vi "Fibonacci - String.vi"(7 "Memo":string[](array[string]), 11 "n":u32) -> (3 "fib(n)":string)   [LabVIEW 2013, in "Problem 25.lvlib"]
uses:
  Problem 25.lvlib
  Problem 20/Problem 20.lvlib
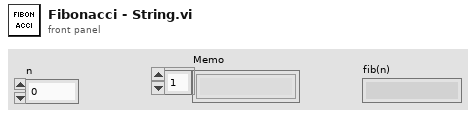
[diagram p1: front panel]
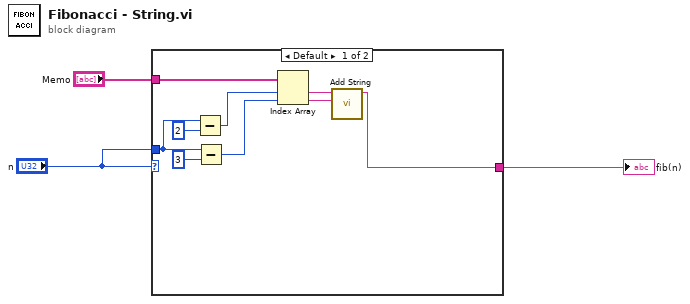
[diagram p0: block diagram]
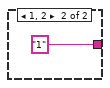
[diagram p2: hidden frame]
diagram:
  n1 = case shown="Default" "n" {
    tunnel: [w4 "1"] -> w3
    tunnel: "n" -> [w11 _]
    tunnel: "Memo" -> [w9 _]
    frame Default {
      n2 = Subtract(x=w11, y=u32 2) -> (x-y=w7:u32)
      n3 = Subtract(x=w11, y=u32 3) -> (x-y=w8:u32)
      n4 = Index Array(array=w9, index #1=w7, index #2=w8) -> (element #1=w6:string, element #2=w5:string)
      n5 = call "Add String.vi"("y"=w5, "x"=w6) -> ("x + y"=w4:string)  [unwired: 9 in]
    }
    frame 1, 2 {
    }
  }
  "fib(n)" <- w3
